vi "GT_ClrSts.vi"(2 "Count":i16, 3 "Axis":T1 items=["Axis Control"=0, "Axis 1"=1, "Axis 2"=2, "Axis 3"=3, "Axis 4"=4, "Axis 5"=5, "Axis 6"=6, "Axis 7"=7, "Axis 8"=8, "Vector Space Control"=16, "Vector Space 1"=17, "Vector Space 2"=18, "Vector Space 3"=19, "Vector Space 4"=20], 4 "rtn_In":cluster{"rtn":i16, "Func":string}) -> (0 "Axis":T1 items=["Axis Control"=0, "Axis 1"=1, "Axis 2"=2, "Axis 3"=3, "Axis 4"=4, "Axis 5"=5, "Axis 6"=6, "Axis 7"=7, "Axis 8"=8, "Vector Space Control"=16, "Vector Space 1"=17, "Vector Space 2"=18, "Vector Space 3"=19, "Vector Space 4"=20], 1 "rtn_Out":cluster{"rtn":i16, "Func":string})   [LabVIEW 2014]
uses:
  <vilib>/Motion/FlexMotion/CustomControls/CustomControls.llb/AxisOrVectorSpaceControl To Control.flx
  VC6/gts.dll
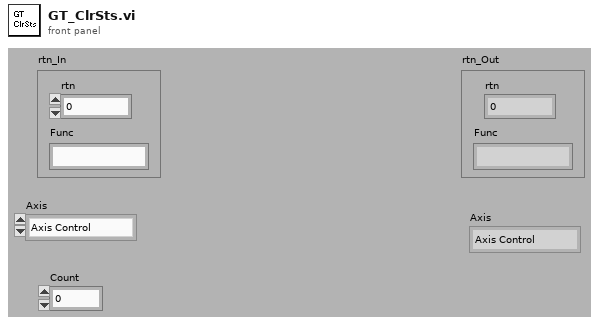
[diagram p1: front panel]
types:
  T1 = typedef "AxisOrVectorSpaceControl To Control.flx" = u16
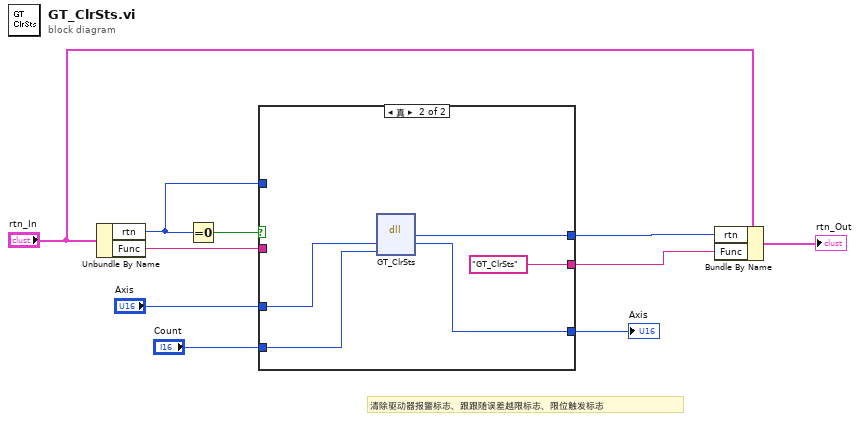
[diagram p0: block diagram]
diagram:
  # "清除驱动器报警标志、跟跟随误差越限标志、限位触发标志"
  n1 = Unbundle By Name("rtn_In") -> ("rtn"=w3:i16, "Func"=w4:string)
  n2 = Equal To 0?(x=w3) -> (x = 0?=w10:bool)
  n3 = case shown="真" w10 {
    tunnel: [w11 w18] -> w7
    tunnel: [w12 "GT_ClrSts" ("Func")] -> w6
    tunnel: "Axis" -> [w13 w16]
    tunnel: "Count" -> [_ w15]
    tunnel: [w13 w14] -> w1
    tunnel: w4 -> [w12 _]
    tunnel: w3 -> [w11 _]
    frame False {
    }
    frame True {
      n4 = dll-call lib="PTH2Fabs DNewGTS AC-800LWin7版源程序-20170926gts85VC6gts.dll" fn="GT_ClrSts"("axis"=w16, "Count"=w15) -> ("rtn"=w18:i16, "axis"=w14:i16)  [unwired: 4 in, 2 out]
    }
  }
  "Axis" <- w1
  n5 = Bundle By Name(cluster="rtn_In", "rtn"=w7, "Func"=w6) -> (→"rtn_Out":cluster{"rtn":i16, "Func":string})
